vi "Fix gRPC Server Dependencies.vi"(8 "error in":errorcluster, 9 "Proto Names":T1, 10 "Project Path":path, 11 "VI Refnum":refnum<vi>) -> (0 "error out":errorcluster)   [LabVIEW 2021, in "Plugin Generator.lvlib"]
uses:
  Plugin Generator.lvlib
  Typedef/Proto Names.ctl
  <vilib>/Utility/traverseref.llb/TRef TravTarget.ctl
  <vilib>/Utility/traverseref.llb/VI Scripting - Traverse.lvlib
  <vilib>/CIF Foundation/CIF LabVIEW Scripting/LV Scripting/LV Scripting Utilities.lvlib
  <vilib>/CIF Foundation/CIF Utilities/File/File_CIF_U.lvlib
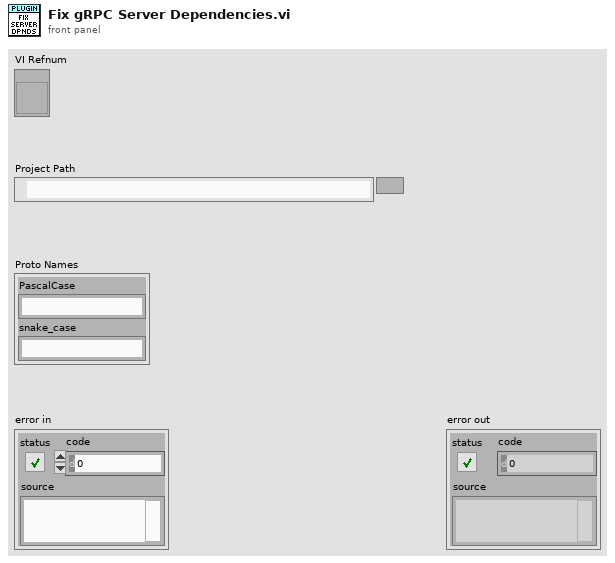
[diagram p1: front panel]
types:
  T1 = typedef "Plugin Generator.lvlib/Proto Names.ctl" = cluster{"PascalCase":string, "snake_case":string}
  T2 = typedef "TRef TravTarget.ctl" = enum16{"FP", "BD", "Other"}
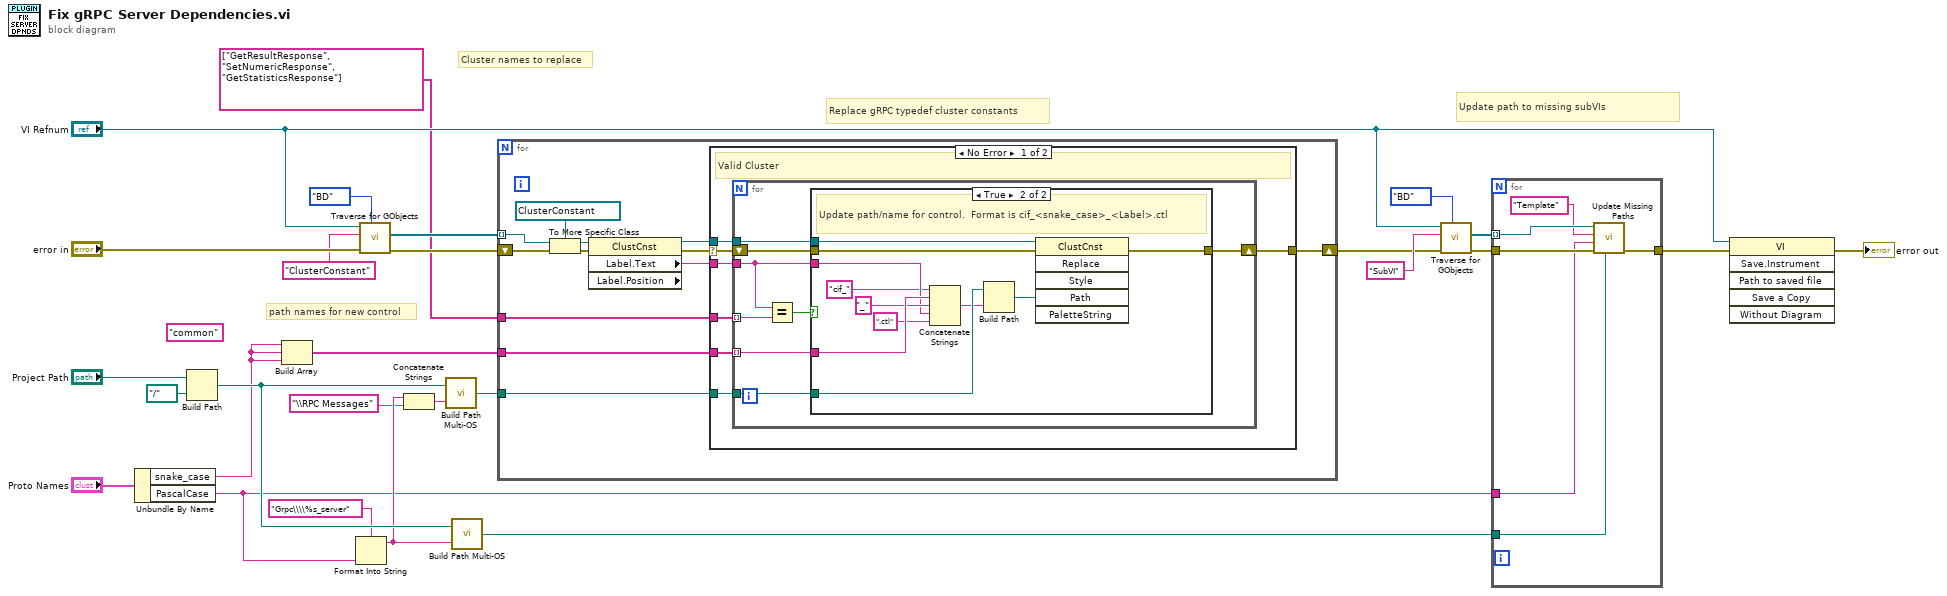
[diagram p0: block diagram]
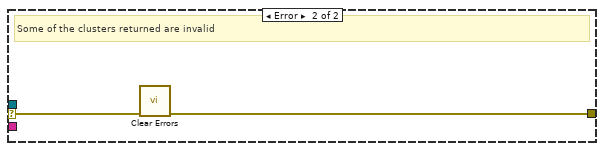
[diagram p3: hidden frame]
diagram:
  (unwired) "common" ("element")
  # "path names for new control"
  # "Cluster names to replace"
  # "Update path to missing subVIs"
  # "Replace gRPC typedef cluster constants"
  n1 = Unbundle By Name("Proto Names") -> ("snake_case"=w1:string, "PascalCase"=w5:string)
  n2 = Build Path(base path="Project Path", name or relative path=path "../..") -> (appended path=w17:path)
  n3 = Build Array(w1, w1, w1) -> (w3:string[])
  n4 = Format Into String(format string="Grpc\\\\%s_server" ("Class Name"), w5) -> (resulting string=w15:string)  [unwired: 2 in, 1 out]
  n5 = call <vilib>:"Traverse for GObjects.vi"("Traverse Target"=TRef_TravTarget."BD", "error in (no error)"="error in", "Class Name"="ClusterConstant", "VI Refnum"="VI Refnum") -> ("error out"=w19:errorcluster, "References"=w23:refnum<vi>[])  [unwired: 4 in, 2 out]
  n6 = Concatenate Strings(w15, "\\RPC Messages" ("Class Name")) -> (w13:string)
  n7 = call <vilib>:"Build Path Multi-OS.vi"("name or relative path"=w13, "base path"=w17) -> ("appended path"=w18:path)
  n8 = call <vilib>:"Build Path Multi-OS.vi"("name or relative path"=w15, "base path"=w17) -> ("appended path"=w4:path)
  n9 = for {
    tunnel: w23 -> [w39] mode=indexing
    shift-right: [w28] -> w7
    shift-left: w19 -> [w34]
    tunnel: w18 -> [w33]
    tunnel: w3 -> [w32]
    tunnel: string[] ["GetResultResponse", "SetNumericResponse", "GetStatisticsResponse"] -> [w31]
    n10 = To More Specific Class(target class=refnum<vi> refnum ("x"), reference=w39, error in=w34) -> (specific class reference=w35:refnum<vi>, error out=w37:errorcluster)
    n11 = property class="ClustCnst" props=["Label", "Text", "Label", "Position"](reference=w35, error in=w37) -> (reference out=w36:refnum<vi>, error out=w29:errorcluster, "Label.Text"=w30:string)  [unwired: 1 out]
    n12 = case shown="No Error" w29 {
      selector: w29 -> [w40 w68]
      tunnel: w36 -> [w46 _]
      tunnel: w33 -> [w45 _]
      tunnel: w32 -> [w44 _]
      tunnel: w31 -> [w43 _]
      tunnel: w30 -> [w42 _]
      tunnel: [w41 w67] -> w28
      frame No Error {
        # "Valid Cluster"
        n13 = for {
          tunnel: w46 -> [w53]
          tunnel: w44 -> [w50] mode=indexing
          tunnel: w42 -> [w47]
          tunnel: w45 -> [w51]
          shift-right: [w52] -> w41
          shift-left: w40 -> [w54]
          tunnel: w43 -> [w49] mode=indexing
          n14 = Equal?(x=w47, y=w49) -> (x = y?=w48:bool)
          n15 = case shown="True" w48 {
            tunnel: w54 -> [w55 w61]
            tunnel: w53 -> [_ w66]
            tunnel: [w55 w56] -> w52
            tunnel: w51 -> [_ w65]
            tunnel: w50 -> [_ w63]
            tunnel: w47 -> [_ w60]
            frame False {
            }
            frame True {
              # "Update path/name for control.  Format is cif_<snake_case>_<Label>.ctl"
              n16 = Concatenate Strings("cif_", w63, "_" ("string"), w60, ".ctl" ("string")) -> (w58:string)
              n17 = Build Path(base path=w65, name or relative path=w58) -> (appended path=w64:path)
              n18 = invoke class="ClustCnst" method="Replace"(reference=w66, error in=w61, "Path"=w64) -> (error out=w56:errorcluster)  [unwired: 3 in, 5 out]
            }
          }
        }
      }
      frame Error {
        # "Some of the clusters returned are invalid"
        n19 = call <vilib>:"Clear Errors.vi"("error in (no error)"=w68) -> ("error out"=w67:errorcluster)  [unwired: 5 in, 1 out]
      }
    }
  }
  n20 = call <vilib>:"Traverse for GObjects.vi"("Traverse Target"=TRef_TravTarget."BD", "error in (no error)"=w7, "Class Name"="SubVI", "VI Refnum"="VI Refnum") -> ("error out"=w9:errorcluster, "References"=w10:refnum<vi>[])  [unwired: 4 in, 2 out]
  n21 = for {
    tunnel: w10 -> [w73] mode=indexing
    tunnel: w5 -> [w72]
    tunnel: w9 -> [w74]
    tunnel: [w71] -> w6
    tunnel: w4 -> [w70]
    n22 = call <vilib>:"Update Missing Paths.vi"("Search Path"=w70, "error in (no error)"=w74, "New Subname"=w72, "Subname to Replace"="Template" ("search string"), "GObject in"=w73) -> ("error out"=w71:errorcluster)  [unwired: 6 in]
  }
  n23 = invoke class="VI" method="Save.Instrument"(reference="VI Refnum", error in=w6) -> (error out=→"error out":errorcluster)  [unwired: 4 in, 5 out]
